vi "Main.vi"(11 "Module Admin":refnum<class "Delacor_lib_QMH_Module Admin.lvclass">) -> ()   [LabVIEW 2023, in "Settings Editor.lvlib"]
doc: "This template is based off of the Queued Message Handler design pattern and the Queued Message Handler project template that ships with LabVIEW.\n\nThe main difference is that the queue is private to this module and communication between modules is performed via Broadcast and Request events.\n\nRequest events are wrapped in public API methods and are handled in the Event Handling Loop (EHL) of this VI. Any module can register for Broadcast events sent by this module. The EHL generates messages based on user interface actions.\n\nThe Message Handling Loop (MHL) processes messages generated by the EHL, or by other messages. The messages are string values, so new messages can be added easily to the Message Cases case structure in the MHL. Each message cluster can also provide an optional value for Message Data, which is a variant that can be converted to whatever message-specific data is required.\n_____\nBased on Delacor QMH Project Template 4.0.0.47.\n_____\nBased on DQMH Project Template 6.1.0.94."
uses:
  Settings Editor.lvlib
  Module Data--cluster.ctl
  <vilib>/Delacor/Delacor QMH/Libraries/Message Queue_class/Delacor_lib_QMH_Message Queue.lvclass
  <vilib>/Delacor/Delacor QMH/Libraries/Message Queue_class/Delacor_lib_QMH_Enqueue Message (Single).vi
  <vilib>/ErrorRing/Error Ring.xnode
  <vilib>/Utility/error.llb/Error Cluster From Error Code.vi
  <vilib>/Delacor/Delacor QMH/Libraries/Module Admin_class/Delacor_lib_QMH_Module Admin.lvclass
  Stop Argument--cluster.ctl
  <vilib>/Utility/miscctls.llb/LVPointTypeDef.ctl
  CML Shared/Signal Type--enum.ctl
  CML Shared/CML Shared.lvlib
  CML Shared/Calibration Values--cluster.ctl
  Update Application Settings (Reply Payload)--cluster.ctl
  Update Application Settings Argument--cluster.ctl
  Settings--cluster.ctl
  test (Reply Payload)--cluster.ctl
  test Argument--cluster.ctl
panel:
  in  "Calibration Values":T1[](array[typedef])
  in  "Cancel":bool
  in  "OK":bool
  in  "Log File Base Path":path
  in  "Signal Type":T2
  out "error out":errorcluster
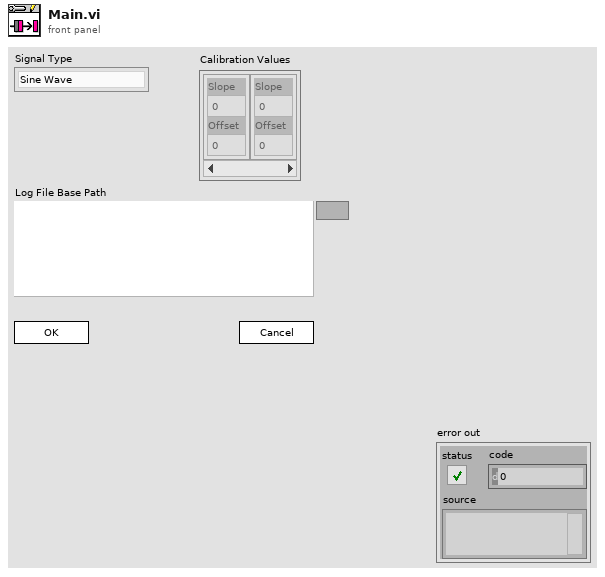
[diagram p1: front panel]
types:
  T1 = typedef "CML Shared.lvlib/Calibration Values--cluster.ctl" = cluster{"Slope":dbl, "Offset":dbl}
  T2 = typedef "CML Shared.lvlib/Signal Type--enum.ctl" = enum16{"Sine Wave", "Square with Noise"}
  T3 = typedef "Settings Editor.lvlib/Request Events--cluster.ctl" = cluster{"Stop Module":refnum<user-event>, "Show Panel":refnum<user-event>, "Hide Panel":refnum<user-event>, "Get Module Execution Status":refnum<user-event>, "Show Diagram":refnum<user-event>, "Update Application Settings":refnum<user-event>, "test":refnum<user-event>}
  T4 = typedef "Settings Editor.lvlib/Module Data--cluster.ctl" = cluster{"Settings":T5}
  T5 = typedef "Settings Editor.lvlib/Settings--cluster.ctl" = cluster{"Signal Type":T2, "Calibration Array":T1[], "Log File Base Path":path}
  T6 = enum32{"invalid lock state", "Not Locked", "Locked (No Password)", "Password-protected"}
  T7 = typedef "Settings Editor.lvlib/Stop Argument--cluster.ctl" = cluster{"Origin":string, "Exit via Stop Module Req?":bool, "Wait for Module to stop?":bool}
  T8 = typedef "Settings Editor.lvlib/Update Application Settings Argument--cluster.ctl" = cluster{"Wait Notifier":refnum<notifier>, "wait for reply":bool}
  T9 = typedef "Settings Editor.lvlib/test Argument--cluster.ctl" = cluster{"Wait Notifier":refnum<notifier>, "wait for reply":bool}
  T10 = typedef "LVPointTypeDef.ctl" = cluster{"Horizontal":i16, "Vertical":i16}
  T11 = enum32{"Invalid", "Standard", "Closed", "Hidden", "Minimized", "Maximized"}
  T12 = typedef "Settings Editor.lvlib/Update Application Settings (Reply Payload)--cluster.ctl" = cluster{"Settings":T5, "error":errorcluster}
  T13 = typedef "Settings Editor.lvlib/test (Reply Payload)--cluster.ctl" = cluster{"Cluster":cluster{"Numeric":dbl, "Numeric 2":dbl, "Numeric 3":dbl, "Numeric 4":dbl, "Numeric 5":dbl}, "error":errorcluster}
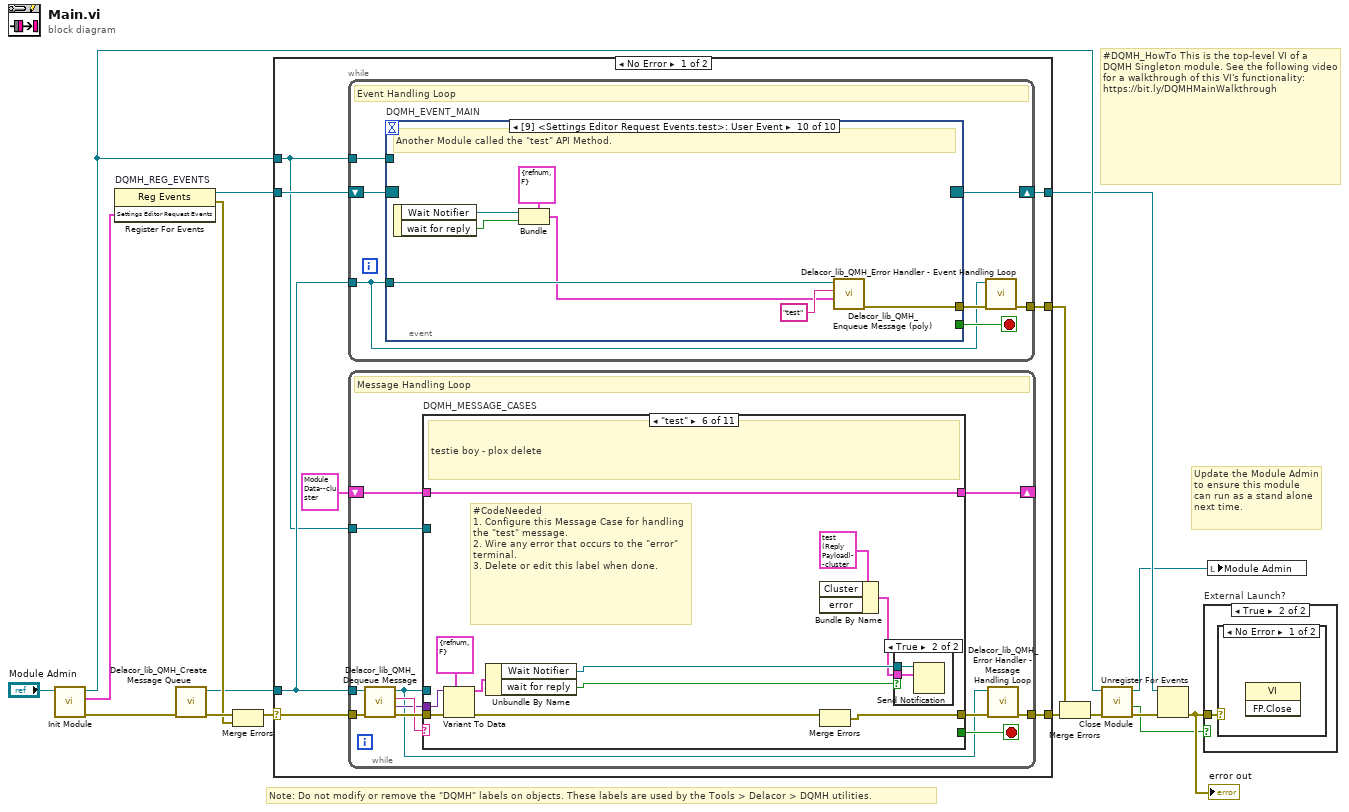
[diagram p0: block diagram]
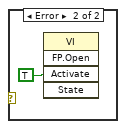
[diagram p3: hidden frame]
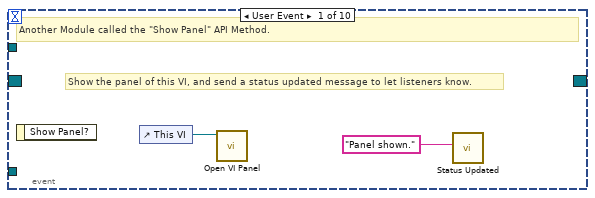
[diagram p4: hidden frame]
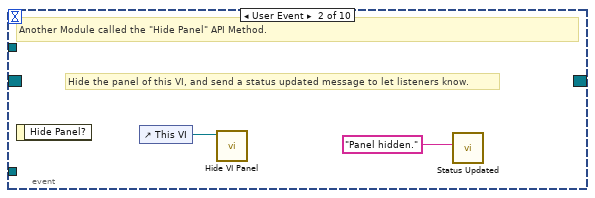
[diagram p5: hidden frame]
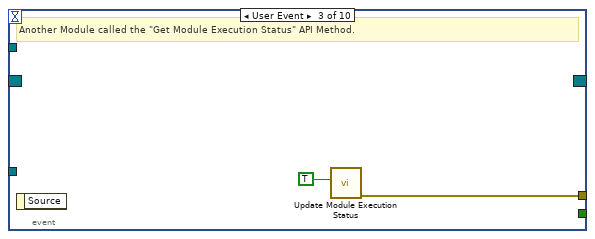
[diagram p6: hidden frame]
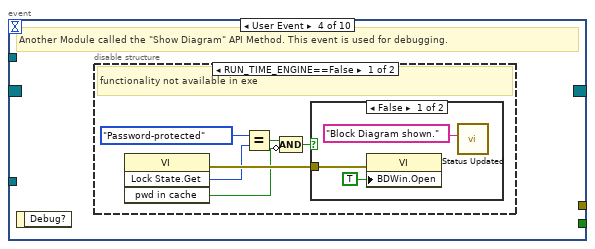
[diagram p7: hidden frame]
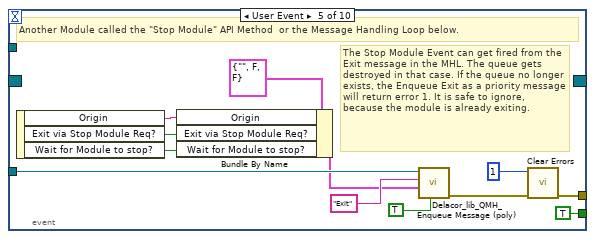
[diagram p10: hidden frame]
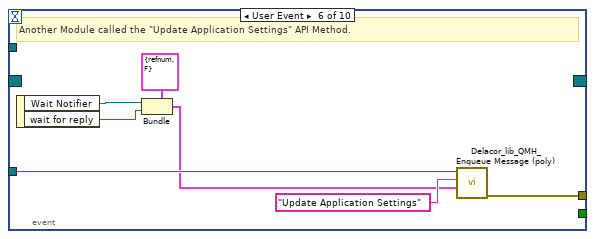
[diagram p11: hidden frame]
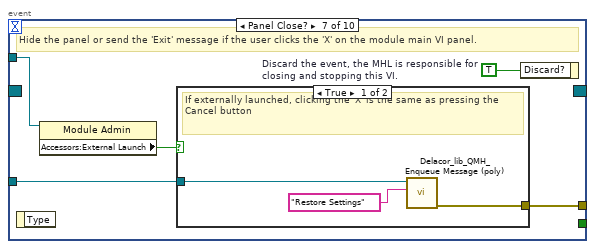
[diagram p12: hidden frame]
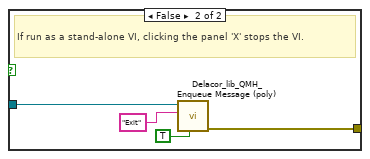
[diagram p13: hidden frame]
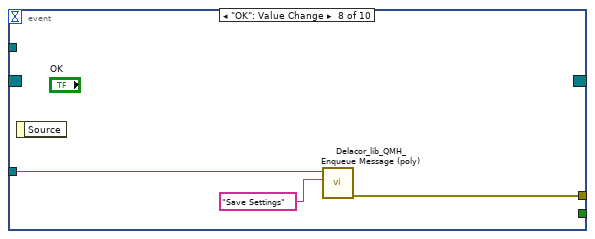
[diagram p14: hidden frame]
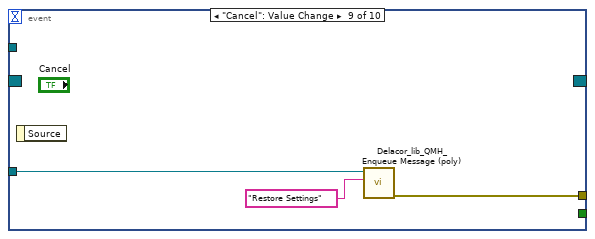
[diagram p15: hidden frame]
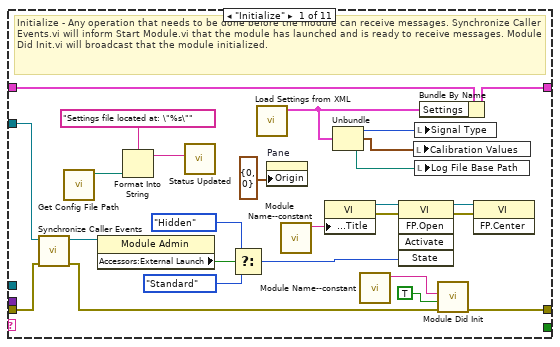
[diagram p16: hidden frame]
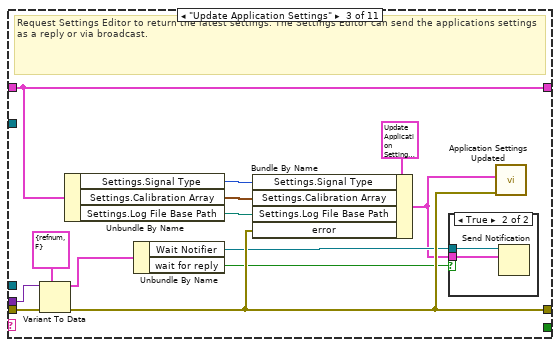
[diagram p18: hidden frame]
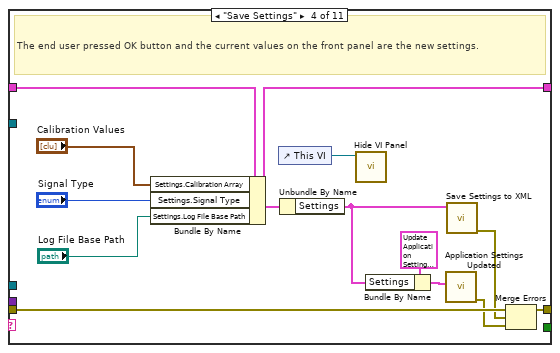
[diagram p20: hidden frame]
diagram:
  # "#DQMH_HowTo This is the top-level VI of a DQMH Singleton module. See the following video for a walkthrough of this VI's functionality: https://bit.ly/DQMHMainWalkthrough"
  # "Note: Do not modify or remove the \"DQMH\" labels on objects. These labels are used by the Tools > Delacor > DQMH utilities."
  # "Update the Module Admin to ensure this module can run as a stand alone next time."
  n1 = call "Init Module.vi"("Singleton Module Admin in"="Module Admin") -> ("error out"=w16:errorcluster, "Settings Editor Request Events"=w5:T3, "Singleton Module Admin out"=w8:refnum<class "Delacor_lib_QMH_Module Admin.lvclass">)  [unwired: 8 in]
  n2 = register-events "DQMH_REG_EVENTS"(w5) -> (reference out=w6:refnum<event-registration>, error out=w9:errorcluster)  [unwired: 2 in]
  n3 = call <vilib>:"Delacor_lib_QMH_Create Message Queue.vi"("error in"=w16) -> ("error out"=w11:errorcluster, "Message Queue"=w4:refnum<class "Delacor_lib_QMH_Message Queue.lvclass">)  [unwired: 9 in]
  n4 = Merge Errors(w11, w9) -> (w10:errorcluster)
  n5 = case shown="No Error" w10 {
    selector: w10 -> [w23 w229]
    tunnel: [w25 w228] -> w17
    tunnel: [w22 w235] -> w7
    tunnel: w6 -> [w20 w235]
    tunnel: w4 -> [w19 w230]
    tunnel: [w24 _] -> w14
    tunnel: w8 -> [w18 w231]
    frame No Error {
      n6 = while {
        tunnel: w19 -> [w26]
        shift-right: [w29] -> w22
        shift-left: w20 -> [w30]
        tunnel: [w31] -> w24
        tunnel: w18 -> [w27]
        stop <- w28 stop-if-true
        # "Event Handling Loop"
        n7 = event "DQMH_EVENT_MAIN" shown="[9] <Settings Editor Request Events.test>: User Event" {
          selector: w30 -> [_ _ _ _ _ _ _ _ _ _]
          dyn-events: [_ _ _ _ _ _ _ _ _ _] -> w29
          timeout: _ -> [_ _ _ _ _ _ _ _ _ _]
          tunnel: [_ _ _ _ TRUE ("Discard?") _ _ _ _ _] -> w28
          tunnel: w26 -> [_ _ _ _ w55 w66 w69 w79 w83 w91]
          tunnel: [_ _ w38 _ w58 w62 w71 w80 w82 w85] -> w32
          tunnel: w27 -> [_ _ _ _ _ _ w68 _ _ _]
          event User Event {
            # "Show the panel of this VI, and send a status updated message to let listeners know."
            # "Another Module called the \"Show Panel\" API Method."
            n8 = event-data() -> ()  [unwired: 1 in, 1 out]
            n9 = control-ref of="This VI"() -> (w34:refnum<vi>)
            n10 = call "Open VI Panel.vi"("VI"=w34) -> ()  [unwired: 10 in, 1 out]
            n11 = call "Status Updated.vi"("Status"="Panel shown." ("format string")) -> ()  [unwired: 10 in, 1 out]
          }
          event User Event {
            # "Hide the panel of this VI, and send a status updated message to let listeners know."
            # "Another Module called the \"Hide Panel\" API Method."
            n12 = event-data() -> ()  [unwired: 1 in, 1 out]
            n13 = control-ref of="This VI"() -> (w36:refnum<vi>)
            n14 = call "Hide VI Panel.vi"("VI"=w36) -> ()  [unwired: 10 in, 1 out]
            n15 = call "Status Updated.vi"("Status"="Panel hidden." ("format string")) -> ()  [unwired: 10 in, 1 out]
          }
          event User Event {
            # "Another Module called the \"Get Module Execution Status\" API Method."
            n16 = event-data() -> ()  [unwired: 1 in, 1 out]
            n17 = call "Update Module Execution Status.vi"("Running?"=TRUE) -> ("error out"=w38:errorcluster)  [unwired: 10 in]
          }
          event User Event {
            # "Another Module called the \"Show Diagram\" API Method. This event is used for debugging."
            n18 = event-data() -> ()  [unwired: 1 in, 1 out]
            n19 = disable-structure shown="RUN_TIME_ENGINE==False" {
              frame condition #0 (active) {
                # "functionality not available in exe"
                n20 = invoke class="VI" method="Lock State.Get"() -> (error out=w44:errorcluster, "Get Lock State"=w43:T6, "pwd in cache"=w40:bool)  [unwired: 4 in, 1 out]
                n21 = Equal?(x=T6."Password-protected", y=w43) -> (x = y?=w41:bool)
                n22 = Compound Arithmetic op=AND(w41, invert w40) -> (w39:bool)
                n23 = case shown="False" w39 {
                  tunnel: w44 -> [w47 _]
                  frame False {
                    n24 = property class="VI"(error in=w47, "BDWin.Open"=TRUE ("Block Diagram Window:Open")) -> ()  [unwired: 1 in, 2 out]
                    n25 = call "Status Updated.vi"("Status"="Block Diagram shown." ("format string")) -> ()  [unwired: 10 in, 1 out]
                  }
                  frame True {
                    # "Password-protected VI, and the password is not in the cache. Do not show the diagram."
                  }
                }
              }
              frame condition #1 {
              }
            }
          }
          event User Event {
            # "The Stop Module Event can get fired from the Exit message in the MHL. The queue gets destroyed in that case. If the queue no longer exists, the Enqueue Exit as a priority message will return error 1. It is safe to ignore, because the module is already exiting."
            # "Another Module called the \"Stop Module\" API Method  or the Message Handling Loop below."
            n26 = event-data() -> ("Origin"=w48:string, "Exit via Stop Module Req?"=w51:bool, "Wait for Module to stop?"=w50:bool)  [unwired: 1 in]
            n27 = Bundle By Name(cluster=T7 {"Origin"="", "Exit via Stop Module Req?"=FALSE, "Wait for Module to stop?"=FALSE} ("Stop Argument"), "Origin"=w48, "Exit via Stop Module Req?"=w51, "Wait for Module to stop?"=w50) -> (w49:T7)
            n28 = call-poly <vilib>:"Delacor_lib_QMH_Enqueue Message (poly).vi"("Priority Message? (F)"=TRUE, "Message Data"=w49, "Message"="Exit", "Message Queue in"=w55) -> ("error out"=w59:errorcluster)  [unwired: 6 in, 1 out]
            n29 = call <vilib>:"Clear Errors.vi"("error in (no error)"=w59, "specific error code to clear (0: all)"=1) -> ("error out"=w58:errorcluster)  [unwired: 4 in, 1 out]
          }
          event User Event {
            # "Another Module called the \"Update Application Settings\" API Method."
            n30 = event-data() -> ("Wait Notifier"=w61:refnum<notifier>, "wait for reply"=w60:bool)  [unwired: 1 in]
            n31 = Bundle(cluster=T8 {"Wait Notifier"=refnum, "wait for reply"=FALSE} ("Update Application Settings Argument"), "Wait Notifier"=w61, "wait for reply"=w60) -> (w63:T8)
            n32 = call-poly <vilib>:"Delacor_lib_QMH_Enqueue Message (poly).vi"("Message Data"=w63, "Message"="Update Application Settings", "Message Queue in"=w66) -> ("error out"=w62:errorcluster)  [unwired: 7 in, 1 out]
          }
          event Panel Close? {
            w70 = TRUE  # Discard the event, the MHL is responsible for closing and stopping this VI.
            # "Hide the panel or send the 'Exit' message if the user clicks the 'X' on the module main VI panel."
            n33 = event-data() -> ()  [unwired: 1 in, 1 out]
            n34 = property class="Module Admin"(reference=w68) -> ("Accessors:External Launch"=w67:bool)  [unwired: 1 in, 2 out]
            n35 = case shown="True" w67 {
              tunnel: w69 -> [w73 w77]
              tunnel: [w72 w78] -> w71
              frame True {
                # "If externally launched, clicking the 'X' is the same as pressing the Cancel button"
                n36 = call-poly <vilib>:"Delacor_lib_QMH_Enqueue Message (poly).vi"("Message"="Restore Settings", "Message Queue in"=w73) -> ("error out"=w72:errorcluster)  [unwired: 8 in, 1 out]
              }
              frame False {
                # "If run as a stand-alone VI, clicking the panel 'X' stops the VI."
                n37 = call-poly <vilib>:"Delacor_lib_QMH_Enqueue Message (poly).vi"("Priority Message? (F)"=TRUE, "Message"="Exit", "Message Queue in"=w77) -> ("error out"=w78:errorcluster)  [unwired: 7 in, 1 out]
              }
            }
            n38 = event-data("Discard?"=w70) -> ()  [unwired: 1 in, 1 out]
          }
          event "OK": Value Change {
            n39 = event-data() -> ()  [unwired: 1 in, 1 out]
            n40 = call-poly <vilib>:"Delacor_lib_QMH_Enqueue Message (poly).vi"("Message"="Save Settings", "Message Queue in"=w79) -> ("error out"=w80:errorcluster)  [unwired: 8 in, 1 out]
          }
          event "Cancel": Value Change {
            n41 = event-data() -> ()  [unwired: 1 in, 1 out]
            n42 = call-poly <vilib>:"Delacor_lib_QMH_Enqueue Message (poly).vi"("Message"="Restore Settings", "Message Queue in"=w83) -> ("error out"=w82:errorcluster)  [unwired: 8 in, 1 out]
          }
          event User Event {
            # "Another Module called the \"test\" API Method."
            n43 = event-data() -> ("Wait Notifier"=w87:refnum<notifier>, "wait for reply"=w86:bool)  [unwired: 1 in]
            n44 = Bundle(cluster=T9 {"Wait Notifier"=refnum, "wait for reply"=FALSE} ("test Argument"), "Wait Notifier"=w87, "wait for reply"=w86) -> (w88:T9)
            n45 = call-poly <vilib>:"Delacor_lib_QMH_Enqueue Message (poly).vi"("Message Data"=w88, "Message"="test", "Message Queue in"=w91) -> ("error out"=w85:errorcluster)  [unwired: 7 in, 1 out]
          }
        }
        n46 = call-dynamic "Delacor_lib_QMH_Error Handler - Event Handling Loop.vi"("error in"=w32, "Message Queue in"=w26) -> ("dup error in"=w31:errorcluster)  [unwired: 8 in, 1 out]
      }
      n47 = while {
        tunnel: w19 -> [w94]
        shift-right: [w98] -> _
        shift-left: T4 {"Settings"={"Signal Type"=enum."Sine Wave", "Calibration Array"=[{"Slope"=1.0, "Offset"=0.0}], "Log File Base Path"=path ""}} ("Data Cluster") -> [w99]
        tunnel: w23 -> [w102]
        tunnel: [w100] -> w25
        tunnel: w18 -> [w92]
        stop <- w97 stop-if-true
        # "Message Handling Loop"
        n48 = call-dynamic "Delacor_lib_QMH_Dequeue Message.vi"("error in"=w102, "Message Queue in"=w94) -> ("error out"=w101:errorcluster, "Message Data"=w95:variant, "Message"=w96:string, "Message Queue out"=w93:refnum<class "Delacor_lib_QMH_Message Queue.lvclass">)  [unwired: 6 in]
        n49 = case "DQMH_MESSAGE_CASES" shown="\"test\"" w96 {
          selector: w96 -> [_ _ _ _ _ _ _ _ _ _ w215]
          tunnel: w93 -> [_ _ _ _ _ _ _ _ w185 w207 _]
          tunnel: w101 -> [w128 w131 w143 w149 w164 w175 w180 w182 w192 w213 w217]
          tunnel: [w126 w131 w144 w150 w164 w165 w179 w182 w188 w210 w218] -> w103
          tunnel: w99 -> [w117 w130 w137 w159 w163 w174 w178 w181 w187 w206 w216]
          tunnel: [w116 w130 w137 w156 w163 w174 w178 w181 w187 w206 w216] -> w98
          tunnel: [_ _ _ _ _ _ _ _ _ w205 _] -> w97
          tunnel: w95 -> [_ _ w142 _ _ w172 _ _ w186 w204 _]
          tunnel: w92 -> [w118 _ _ _ _ _ _ _ w184 w199 _]
          frame "Initialize" {
            # "Initialize - Any operation that needs to be done before the module can receive messages. Synchronize Caller Events.vi will inform Start Module.vi that the module has launched and is ready to receive messages. Module Did Init.vi will broadcast that the module initialized."
            n50 = call "Synchronize Caller Events.vi"("error in (no error)"=w128, "Singleton Module Admin in"=w118) -> ("error out"=w127:errorcluster, "Singleton Module Admin out"=w113:refnum<class "Delacor_lib_QMH_Module Admin.lvclass">)  [unwired: 8 in]
            n51 = call "Get Config File Path.vi"() -> ("XML File Path"=w110:path)  [unwired: 10 in, 1 out]
            n52 = property class="Module Admin"(reference=w113) -> ("Accessors:External Launch"=w122:bool)  [unwired: 1 in, 2 out]
            n53 = Format Into String(format string="Settings file located at: \"%s\"", w110) -> (resulting string=w109:string)  [unwired: 2 in, 1 out]
            n54 = call "Status Updated.vi"("Status"=w109) -> ()  [unwired: 10 in, 1 out]
            n55 = Select(t=T11."Hidden" ("State"), s=w122, f=T11."Standard" ("State")) -> (s? t:f=w119:T11)
            n56 = call "Load Settings from XML.vi"() -> ("Settings out"=w107:T5)  [unwired: 10 in, 1 out]
            n57 = property on="Pane" class="Pane"("Origin"=T10 {"Horizontal"=0, "Vertical"=0}) -> ()  [unwired: 2 in, 2 out]
            n58 = call "Module Name--constant.vi"() -> ("Module Name"=w125:string)  [unwired: 11 in]
            n59 = property class="VI"("Front Panel.Title"=w125) -> (reference out=w124:refnum<vi>, error out=w111:errorcluster)  [unwired: 2 in]
            n60 = Unbundle(w107) -> ("Signal Type"=w106:T2, "Calibration Array"=w105:T1[], "Log File Base Path"=w104:path)
            n61 = call "Module Name--constant.vi"() -> ("Module Name"=w114:string)  [unwired: 11 in]
            n62 = invoke class="VI" method="FP.Open"(reference=w124, error in=w111, "State"=w119) -> (reference out=w123:refnum<vi>, error out=w129:errorcluster)  [unwired: 2 in, 3 out]
            n63 = local write "Calibration Values"(w105) -> ()
            n64 = local write "Signal Type"(w106) -> ()
            n65 = local write "Log File Base Path"(w104) -> ()
            n66 = Bundle By Name(cluster=w117, "Settings"=w107) -> (w116:T4)
            n67 = call "Module Did Init.vi"("error in (no error)"=w127, "Initialized?"=TRUE, "Origin"=w114) -> ("error out"=w126:errorcluster)  [unwired: 8 in]
            n68 = invoke class="VI" method="FP.Center"(reference=w123, error in=w129) -> ()  [unwired: 1 in, 3 out]
          }
          frame "---Module Specific---" {
            # "Separator -- The following cases handle messages specific to this Module."
          }
          frame "Update Application Settings" {
            # "Request Settings Editor to return the latest settings. The Settings Editor can send the applications settings as a reply or via broadcast."
            n69 = Variant To Data(error in=w143, type=T8 {"Wait Notifier"=refnum, "wait for reply"=FALSE} ("Update Application Settings Argument"), Variant=w142) -> (data=w140:T8, error out=w144:errorcluster)
            n70 = Unbundle By Name(w137) -> ("Settings.Signal Type"=w135:T2, "Settings.Calibration Array"=w134:T1[], "Settings.Log File Base Path"=w133:path)
            n71 = Unbundle By Name(w140) -> ("Wait Notifier"=w139:refnum<notifier>, "wait for reply"=w138:bool)
            n72 = Bundle By Name(cluster=T12 {"Settings"={"Signal Type"=enum."Sine Wave", "Calibration Array"=[], "Log File Base Path"=path ""}, "error"={"status"=FALSE, "code"=0, "source"=""}} ("Update Application Settings (Reply Payload)"), "Settings.Signal Type"=w135, "Settings.Calibration Array"=w134, "Settings.Log File Base Path"=w133, "error"=w144) -> (w132:T12)
            n73 = case shown="True" w138 {
              tunnel: w139 -> [_ w146]
              tunnel: w132 -> [_ w145]
              frame False {
              }
              frame True {
                n74 = Send Notification(notification=w145, notifier=w146) -> ()  [unwired: 1 in, 2 out]
              }
            }
            n75 = call "Application Settings Updated.vi"("error in (no error)"=w144, "Reply Payload"=w132) -> ()  [unwired: 9 in, 1 out]
          }
          frame "Save Settings" {
            # "The end user pressed OK button and the current values on the front panel are the new settings."
            n76 = Bundle By Name(cluster=w159, "Settings.Calibration Array"="Calibration Values", "Settings.Signal Type"="Signal Type", "Settings.Log File Base Path"="Log File Base Path") -> (w156:T4)
            n77 = control-ref of="This VI"() -> (w157:refnum<vi>)
            n78 = Unbundle By Name(w156) -> ("Settings"=w151:T5)
            n79 = call "Hide VI Panel.vi"("VI"=w157) -> ()  [unwired: 10 in, 1 out]
            n80 = Bundle By Name(cluster=T12 {"Settings"={"Signal Type"=enum."Sine Wave", "Calibration Array"=[], "Log File Base Path"=path ""}, "error"={"status"=FALSE, "code"=0, "source"=""}} ("Reply Payload"), "Settings"=w151) -> (w152:T12)
            n81 = call "Application Settings Updated.vi"("Reply Payload"=w152) -> ("error out"=w147:errorcluster)  [unwired: 10 in]
            n82 = call "Save Settings to XML.vi"("Settings"=w151) -> ("error out"=w148:errorcluster)  [unwired: 10 in]
            n83 = Merge Errors(w149, w148, w147) -> (w150:errorcluster)
          }
          frame "Restore Settings" {
            # "The end user pressed Cancel button, need to restore the current stored values for the controls on the front panel. No need to broadcast that the settings changed."
            n84 = Unbundle By Name(w163) -> ("Settings.Signal Type"=w162:T2, "Settings.Log File Base Path"=w161:path)
            n85 = local write "Signal Type"(w162) -> ()
            n86 = local write "Log File Base Path"(w161) -> ()
            n87 = control-ref of="This VI"() -> (w160:refnum<vi>)
            n88 = call "Hide VI Panel.vi"("VI"=w160) -> ()  [unwired: 10 in, 1 out]
          }
          frame "test" {
            # "#CodeNeeded\n1. Configure this Message Case for handling the \"test\" message.\n2. Wire any error that occurs to the \"error\" terminal.\n3. Delete or edit this label when done."
            # "testie boy - plox delete"
            n89 = Variant To Data(error in=w175, type=T9 {"Wait Notifier"=refnum, "wait for reply"=FALSE} ("test Argument"), Variant=w172) -> (data=w170:T9, error out=w173:errorcluster)
            n90 = Unbundle By Name(w170) -> ("Wait Notifier"=w169:refnum<notifier>, "wait for reply"=w168:bool)
            n91 = Bundle By Name(cluster=T13 {"Cluster"={"Numeric"=0.0, "Numeric 2"=0.0, "Numeric 3"=0.0, "Numeric 4"=0.0, "Numeric 5"=0.0}, "error"={"status"=FALSE, "code"=0, "source"=""}} ("test (Reply Payload)")) -> (w167:T13)  [unwired: 2 in]
            n92 = Merge Errors(w173) -> (w165:errorcluster)  [unwired: 1 in]
            n93 = case "DQMH_FIRE_NOTIFIER" shown="True" w168 {
              tunnel: w169 -> [_ w177]
              tunnel: w167 -> [_ w176]
              frame False {
              }
              frame True {
                n94 = Send Notification(notification=w176, notifier=w177) -> ()  [unwired: 1 in, 2 out]
              }
            }
          }
          frame "---Copy This Frame---" {
            # "Duplicate this frame when creating new messages.  Change this comment in the duplicated frame to describe this message."
            n95 = Merge Errors(w180) -> (w179:errorcluster)
          }
          frame "---Exit and Error Handling---" {
            # "Separator - The following cases handle errors and exit messages."
          }
          frame "Error" {
            # "Error - Check the error message data and respond accordingly. This message is sent by the \"Error Handler\" VIs at the end of each loop in this application."
            n96 = property class="Module Admin"(reference=w184) -> ("Accessors:External Launch"=w183:bool)  [unwired: 1 in, 2 out]
            n97 = Variant To Data(error in=w192, type=errorcluster {"status"=FALSE, "code"=0, "source"=""} ("error constant"), Variant=w186) -> (data=w193:errorcluster, error out=w190:errorcluster)
            n98 = call "Error Reported.vi"("Error"=w193) -> ()  [unwired: 10 in, 1 out]
            n99 = case shown="False" w183 {
              tunnel: [w198 _] -> w189
              tunnel: w185 -> [w196 _]
              tunnel: w193 -> [w197 _]
              frame False {
                # "If the module is running standalone, then pop up an error dialog and call the \"Exit\" message."
                n100 = call <vilib>:"Simple Error Handler.vi"("error in (no error)"=w197) -> ()  [unwired: 4 in, 5 out]
                n101 = call-poly <vilib>:"Delacor_lib_QMH_Enqueue Message (poly).vi"("Priority Message? (F)"=TRUE, "Message"="Exit", "Message Queue in"=w196) -> ("error out"=w198:errorcluster)  [unwired: 7 in, 1 out]
              }
              frame True {
                # "If the module was launched externally, calling the Error Reported broadcast VI is the only action performed by the \"Error\" message. The module's caller can then process the error appropriately."
              }
            }
            n102 = Merge Errors(w190, w189) -> (w188:errorcluster)
            n103 = local write "error out"(w188) -> ()
          }
          frame "Exit" {
            w203 = 91  # 91: not all Exit messages will have an argument
            w205 = TRUE  # Stop the VI
            # "Release the message queue reference"
            # "Exit - Exit the application."
            n104 = Variant To Data(error in=w213, type=T7 {"Origin"="", "Exit via Stop Module Req?"=FALSE, "Wait for Module to stop?"=FALSE} ("Stop Argument"), Variant=w204) -> (data=w201:T7, error out=w209:errorcluster)
            n105 = call <vilib>:"Clear Errors.vi"("error in (no error)"=w209, "specific error code to clear (0: all)"=w203) -> ("error out"=w212:errorcluster)  [unwired: 4 in, 1 out]
            n106 = control-ref of="This VI"() -> (w200:refnum<vi>)
            n107 = call-dynamic "Delacor_lib_QMH_Release Message Queue.vi"("error in"=w212, "Message Queue"=w207) -> ("error out"=w211:errorcluster)  [unwired: 9 in]
            n108 = call "Handle Exit.vi"("Stop Argument"=w201, "Admin in"=w199, "VI reference"=w200) -> ("error out"=w208:errorcluster)  [unwired: 7 in, 1 out]
            n109 = Merge Errors(w211, w208) -> (w210:errorcluster)
          }
          frame Default {
            # "'Default' case only runs if there is a message that isn't defined in any of the other cases.  Output a programming error."
            n110 = call "Module Name--constant.vi"() -> ("Module Name"=w214:string)  [unwired: 11 in]
            n111 = xnode "Error Ring"("parameter 0"=w215, "parameter 1"=w214) -> ("error out"=w219:errorcluster)
            n112 = Merge Errors(w217, w219) -> (w218:errorcluster)
          }
        }
        n113 = call-dynamic "Delacor_lib_QMH_Error Handler - Message Handling Loop.vi"("error in"=w103, "Message Queue in"=w93) -> ("dup error in"=w100:errorcluster)  [unwired: 8 in, 1 out]
      }
    }
    frame Error {
      # "Synchronize Caller Events.vi will inform Start Module.vi that the module has launched and will let the code calling Start Module.vi register for broadcasts and would permit the caller receive the broadcast that an error occurred at launch time."
      n114 = call "Synchronize Caller Events.vi"("Singleton Module Admin in"=w231) -> ("error out"=w236:errorcluster)  [unwired: 9 in, 1 out]
      n115 = call-dynamic "Delacor_lib_QMH_Release Message Queue.vi"("error in"=w229, "Message Queue"=w230) -> ("error out"=w228:errorcluster)  [unwired: 9 in]
      n116 = call "Module Name--constant.vi"() -> ("Module Name"=w234:string)  [unwired: 11 in]
      n117 = Format Into String(format string="An error occurred during initialization. %s is no longer running.", w234) -> (resulting string=w232:string)  [unwired: 2 in, 1 out]
      n118 = Merge Errors(w228, w236) -> (w237:errorcluster)
      n119 = call "Error Reported.vi"("Additional Information"=w232, "Error"=w237) -> ()  [unwired: 9 in, 1 out]
    }
  }
  n120 = Merge Errors(w14, w17) -> (w13:errorcluster)
  n121 = call "Close Module.vi"("error in (no error)"=w13, "Module Admin in"=w8) -> ("error out"=w15:errorcluster, "External Launch"=w1:bool, "Module Admin out"=w2:refnum<class "Delacor_lib_QMH_Module Admin.lvclass">)  [unwired: 7 in]
  n122 = Unregister For Events(event registration refnum=w7, error in=w15) -> (error out=w12:errorcluster)
  "error out" <- w12
  n123 = case "External Launch?" shown="True" w1 {
    tunnel: w12 -> [_ w238]
    frame False {
    }
    frame True {
      n124 = case shown="No Error" w238 {
        frame No Error {
          n125 = invoke class="VI" method="FP.Close"() -> ()  [unwired: 3 in, 3 out]
        }
        frame Error {
          n126 = invoke class="VI" method="FP.Open"("Activate"=TRUE ("Activate?")) -> ()  [unwired: 4 in, 5 out]
        }
      }
    }
  }
  n127 = local write "Module Admin"(w2) -> ()
